vi "FITS - Save a Single I32 Image to FITS.vi"(5 "Neo Info":T1={"Handle"=104, "Pixel Encoding"="Mono16", "AOI Width"=2560, "AOI Height"=2160, "AOI Stride"=5136, "Row Readout Time"=9.371428571428572e-06, "Frame Readout Time"=0.010121142857142858, "Interframe Time"=8.434285714285715e-05, "Semaphore"=refnum, "SerialNumber"="SCC-02209", "Camera Model"="DC-152Q-C00-FI", "Controller ID"="3", "Firmware Version"="13.8.26.122", "Shutter"="Global", "BDiv"=1, "Time at Synch"=timestamp(3029526000.379448 s since 1904-01-01), "Idx"=0, "PreAmp"="", "Binning"=enum."1x1", "PixelReadoutRate"="", "Exposure (s)"=0.05, "Image Bytes"=11098896, "Image Pixels"=5529600, "SpuriousNoiseFilter"=FALSE, "Overlap"=FALSE, "CycleMode"=""} {"Exposure (s)" format="%^.3g"; "Time at Synch" format="%<%H:%M:%S>T"; "Interframe Time" format="%#_3g"; "Frame Readout Time" format="%_3g"; "Row Readout Time" format="%_3g"}, 6 "byte order (0:big-endian, network order)":T4(ring), 7 "FITS Header":T5={"Wavelength (nm)"=530.15, "Exposure (s)"=0.05, "Tuning Delay (ms)"=1000.0, "Beam Type (-1/1)"=1.0, "Tuning Voltages"=[1.111, 2.222, 3.333, 4.444], "Observer"="observer", "Light Shapping Diffuser"=enum."In Beam", "Comment"="", "Data Type"=9, "Mod Cycles"=0, "SCD Calibration Optics"=enum."1 - Polarizer @0, I+Q", "SCD Emission Line Filter"=enum."1-557.6nm", "Cookbook"="", "COMP-S Calibration Wheel"=enum."Dark", "COMP-S Andover Filter Wheel"=enum."530.3nm/HWB 0.34nm (Fe XIV)", "FOV Rotation (deg)"=66.0, "Objective Lens Position (mm)"=0.0, "Occulter size"=0.0, "Time End"=timestamp(3382374145.421875 s since 1904-01-01), "Acc Exposure (s)"=0.0, "Time Stamp Array"=[], "Camera Serial Number"=[], "Camera Temp"=[], "Camera PI (mm)"=[0.0, 0.0, 0.0], "Time Start"=timestamp(3382374145.421875 s since 1904-01-01), "Peripherals"={"ILX controler"=FALSE, "Zone temperatures"=FALSE, "Andor"=FALSE, "Andor 2"=FALSE, "PI Stages"=FALSE, "AISAS mechanisms"=FALSE, "AISAS Mech.lvclass"=refnum, "Zone temp ref"=variant, "FWs"=FALSE}, "FITS paths"=[], "Cameras"=enum."Andor", "load preset cbk"=FALSE, "periodic check count"=0} {"Camera PI (mm)" format="%_3g"; "Acc Exposure (s)" format="%^.3g"; "Occulter size" format="%.2f"; "Objective Lens Position (mm)" min=70.0 max=152.0 format="%.2f"; "FOV Rotation (deg)" format="%.1f"; "Data Type" items=["LIVE", "DARK", "FLAT", "CALI", "OBSE", "ABSO", "AURE", "TARG", "OBJE", "HOLE", "OREX", "THRO", "CHIP"]; "Exposure (s)" format="%^.3g"; "Wavelength (nm)" format="%_6g"}, 8 "error in":errorcluster, 9 "I32 Image Data":i32[](array[numeric]), 10 "Image #":i32, 11 "FITS File Path":path=path "G:/SCD Data/Level-0/20141030/20141030.160747.FTS") -> (0 "error out":errorcluster, 3 "FITS Path Out":path=path "G:/SCD Data/Level-0/20141030/20141030.160747.FTS")   [LabVIEW 2014]
doc: "Duplicate first measurement\nand put it in first element of\nmeasurement array. This\nis a dummy measurement for the\nprimary header. This is because\nwe don't want any images associated\nwith the primary HDU, just the \nextensions. In the Make FITS\nHeaders VI, the NAXIS is set to 0 in\nthis primary HDU"
uses:
  Controls/SCD - FITS Cluster.ctl
  AISAS/Mech/AISAS Mech.lvclass
  AISAS/Controls/Diffuser.ctl
  Controls/SCD - Calibration Optics Filter Wheel.ctl
  Controls/SCD - EDT - Emission Line Filter Wheel.ctl
  Controls/CoMP-S Controls/Polarization Optics Filter Wheel.ctl
  Controls/CoMP-S Controls/Emission Line Filter Wheel.ctl
  AISAS/Controls/focus.ctl
  Controls/peripherals.ctl
  Controls/Cameras select.ctl
  Camera/Andor Neo Info.ctl
  Controls/beaning.ctl
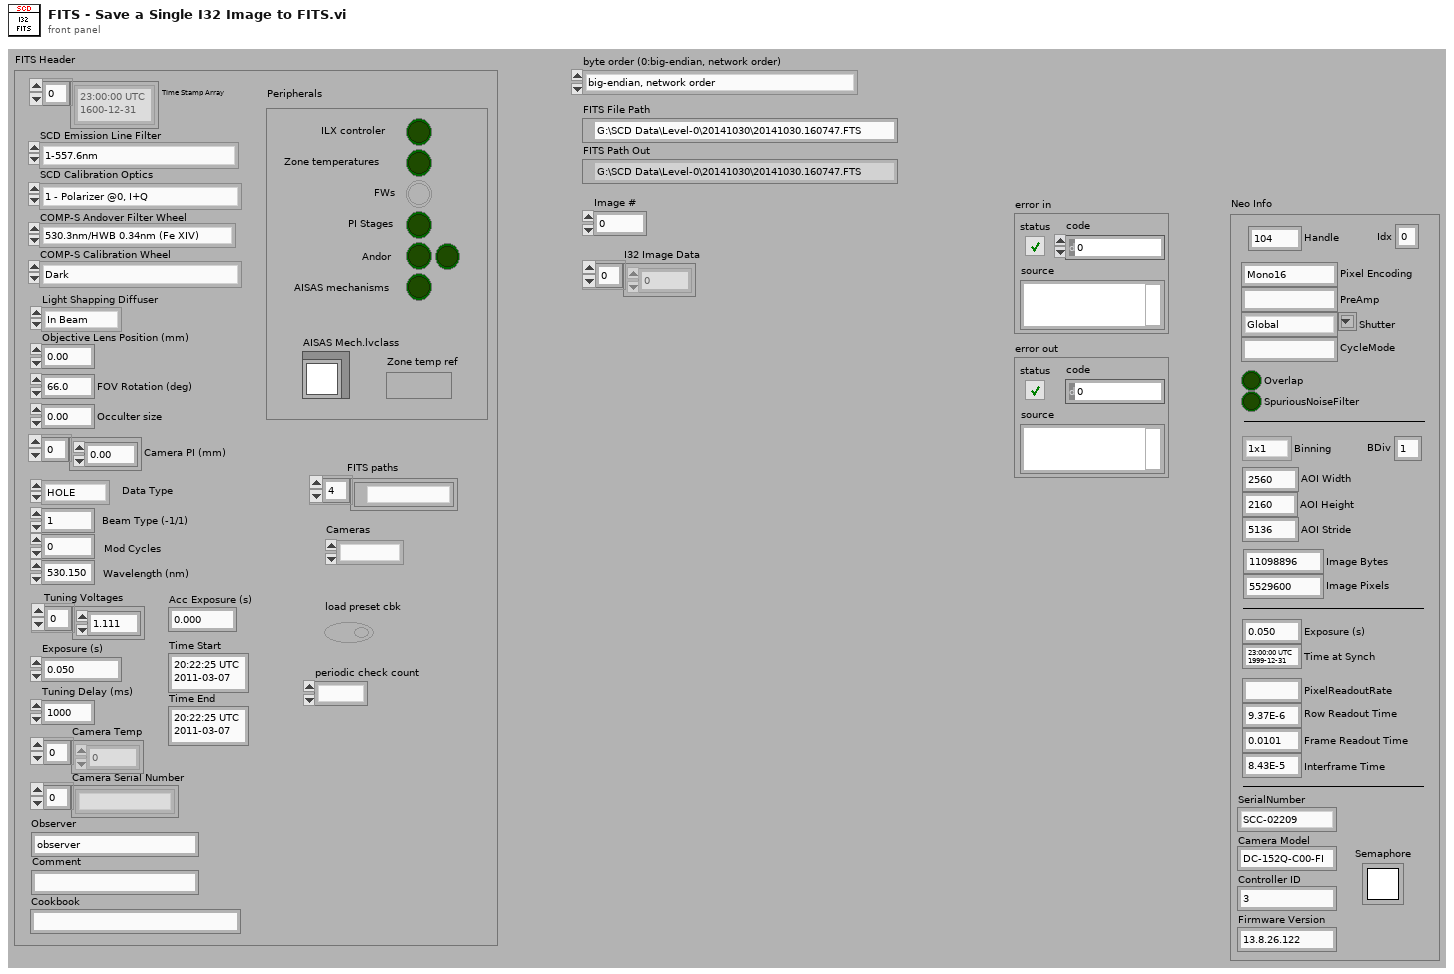
[diagram p1: front panel]
types:
  T1 = typedef "Andor Neo Info.ctl" = cluster{"Handle":i32, "Pixel Encoding":string, "AOI Width":i32, "AOI Height":i32, "AOI Stride":i32, "Row Readout Time":dbl, "Frame Readout Time":dbl, "Interframe Time":dbl, "Semaphore":T2, "SerialNumber":string, "Camera Model":string, "Controller ID":string, "Firmware Version":string, "Shutter":string, "BDiv":u8, "Time at Synch":timestamp, "Idx":i32, "PreAmp":string, "Binning":T3, "PixelReadoutRate":string, "Exposure (s)":dbl, "Image Bytes":i64, "Image Pixels":i64, "SpuriousNoiseFilter":bool, "Overlap":bool, "CycleMode":string}
  T2 = typedef "Semaphore RefNum" = refnum<k1>
  T3 = typedef "beaning.ctl" = enum16{"1x1", "2x2", "3x3", "4x4", "8x8"}
  T4 = enum16{"big-endian, network order", "native, host order", "little-endian"}
  T5 = typedef "SCD - FITS Cluster.ctl" = cluster{"Wavelength (nm)":dbl, "Exposure (s)":dbl, "Tuning Delay (ms)":dbl, "Beam Type (-1/1)":dbl, "Tuning Voltages":dbl[], "Observer":string, "Light Shapping Diffuser":T6, "Comment":string, "Data Type":u16, "Mod Cycles":u16, "SCD Calibration Optics":T7, "SCD Emission Line Filter":T8, "Cookbook":string, "COMP-S Calibration Wheel":T9, "COMP-S Andover Filter Wheel":T10, "FOV Rotation (deg)":dbl, "Objective Lens Position (mm)":T11, "Occulter size":dbl, "Time End":timestamp, "Acc Exposure (s)":dbl, "Time Stamp Array":timestamp[], "Camera Serial Number":string[], "Camera Temp":dbl[], "Camera PI (mm)":dbl[], "Time Start":timestamp, "Peripherals":T12, "FITS paths":path[], "Cameras":T13, "load preset cbk":bool, "periodic check count":i32}
  T6 = typedef "Diffuser.ctl" = enum16{"Out of Beam", "In Beam"}
  T7 = typedef "SCD - Calibration Optics Filter Wheel.ctl" = enum16{"1 - Polarizer @0, I+Q", "2 - Polarizer @90, I-Q", "3 - Polarizer @45, I+U", "4 - Polarizer @135, I-U", "5 - Polarizer @0, Retarder @45, I+V", "6 - Polarizer @0, Retarder @135, I-V", "7 - Dark", "8 - Clear", "9 - N/A"}
  T8 = typedef "SCD - EDT - Emission Line Filter Wheel.ctl" = enum16{"1-557.6nm", "2-587.6nm", "3-589.6nm", "4-630.2nm", "5-656.4nm", "6-849.8nm", "7-854.2nm", "8-866.2nm", "9-1083.0nm"}
  T9 = typedef "Polarization Optics Filter Wheel.ctl" = enum16{"Dark", "Clear", "Exchange Lens", "Polarizer @0, I+Q", "Polarizer @90, I-Q", "Polarizer @45, I+U", "Polarizer @135, I-U", "Polarizer @0, Retarder @45, I+V", "Polarizer @0, Retarder @135, I-V"}
  T10 = typedef "Emission Line Filter Wheel.ctl" = enum16{"530.3nm/HWB 0.34nm (Fe XIV)", "587.6nm/HBW 0.44nm (He I D3)", "637.5nm/HBW 0.53nm (Fe X)", "656.3nm/HBW 0.57nm (H-Alpha)", "789.2nm/HBW 0.85nm (Fe XI)", "854.2nm/HBW 1.01nm (Ca I)", "1074.7nm/HBW 2.34nm (Fe XIII)", "1079.8nm/HBW 1.64nm (Fe XIII)", "1083.0nm/HBW 1.66nm (He I)"}
  T11 = typedef "focus.ctl" = dbl
  T12 = typedef "peripherals.ctl" = cluster{"ILX controler":bool, "Zone temperatures":bool, "Andor":bool, "Andor 2":bool, "PI Stages":bool, "AISAS mechanisms":bool, "AISAS Mech.lvclass":refnum<class "AISAS Mech.lvclass">, "Zone temp ref":variant, "FWs":bool}
  T13 = typedef "Cameras select.ctl" = enum16{"Andor", "GDR"}
  T14 = enum16{"open", "replace", "create", "open or create", "replace or create", "replace or create with confirmation"}
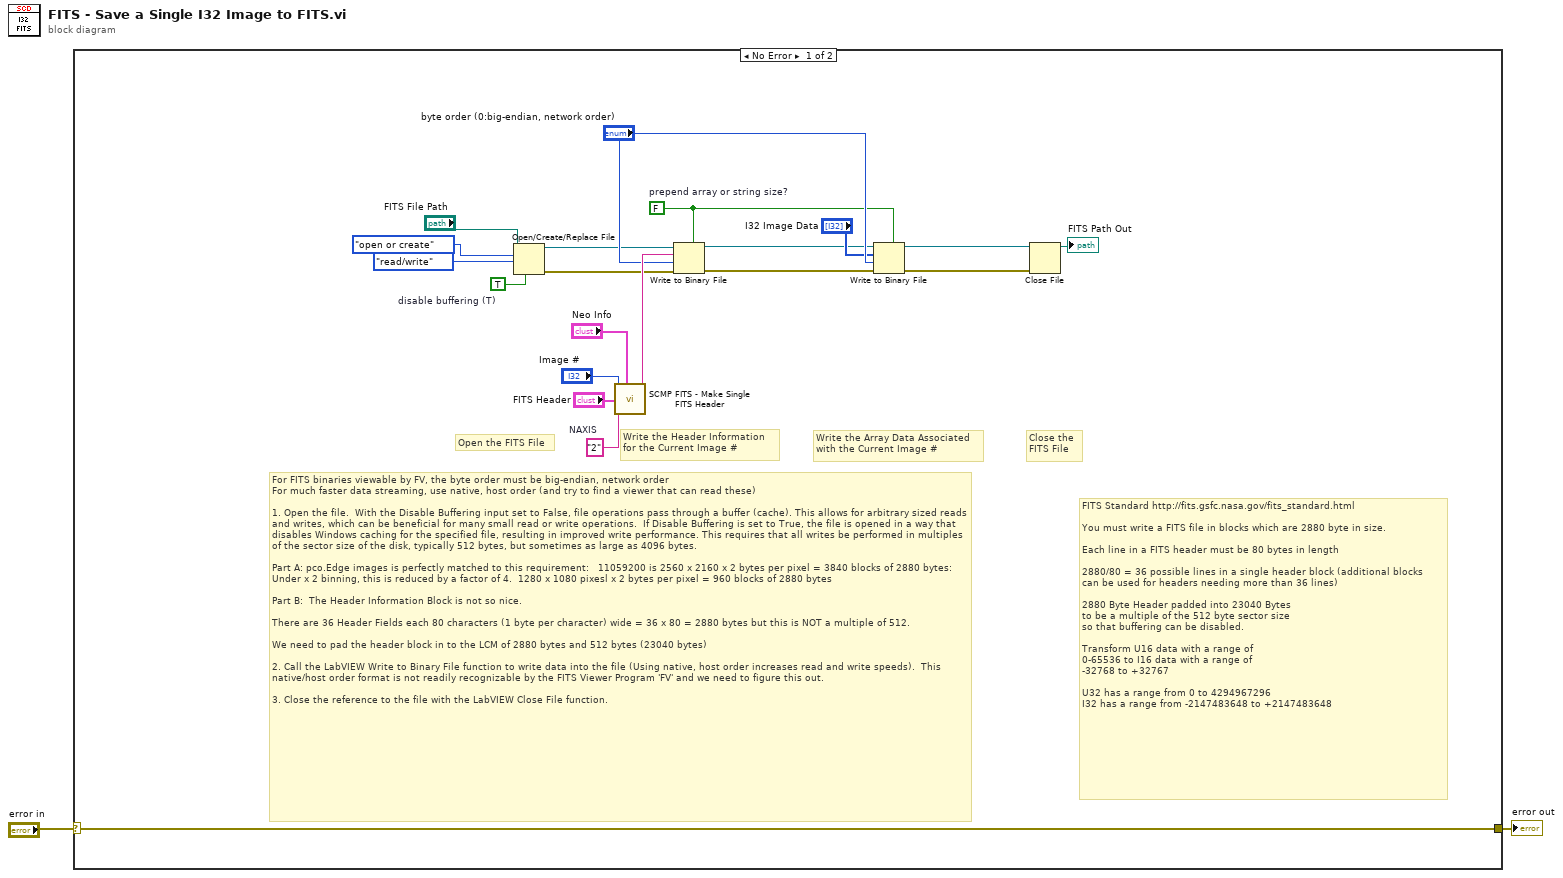
[diagram p0: block diagram]
diagram:
  n1 = case shown="No Error" "error in" {
    selector: "error in" -> [w13 w23]
    tunnel: [w13 w23] -> w1
    frame No Error {
      w4 = "2"  # NAXIS
      w5 = FALSE  # prepend array or string size?
      w15 = TRUE  # disable buffering (T)
      # "FITS Standard http://fits.gsfc.nasa.gov/fits_standard.html\n\nYou must write a FITS file in blocks which are 2880 byte in size.\n\nEach line in a FITS header must be 80 bytes in length\n\n2880/80 = 36 possible lines in a single header block (additional blocks\ncan be used for headers needing more than 36 lines)\n\n2880 Byte Header padded into 23040 Bytes\nto be a multiple of the 512 byte sector size\nso that buffering can be disabled.\n\nTransform U16 data with a range of\n0-65536 to I16 data with a range of\n-32768 to +32767\n\nU32 has a range from 0 to 4294967296\nI32 has a range from -2147483648 to +2147483648"
      # "For FITS binaries viewable by FV, the byte order must be big-endian, network order\nFor much faster data streaming, use native, host order (and try to find a viewer that can read these)\n\n1. Open the file.  With the Disable Buffering input set to False, file operations pass through a buffer (cache). This allows for arbitrary sized reads and writes, which can be beneficial for many small read or write operations.  If Disable Buffering is set to True, the file is opened in a way that disables Windows caching for the specified file, resulting in improved write performance. This requires that all writes be performed in multiples of the sector size of the disk, typically 512 bytes, but sometimes as large as 4096 bytes.\n\nPart A: pco.Edge images is perfectly matched to this requirement:   11059200 is 2560 x 2160 x 2 bytes per pixel = 3840 blocks of 2880 bytes:  Under x 2 binning, this is reduced by a factor of 4.  1280 x 1080 pixesl x 2 bytes per pixel = 960 blocks of 2880 bytes\n\nPart B:  The Header Information Block is not so nice.  \n\nThere are 36 Header Fields each 80 characters (1 byte per character) wide = 36 x 80 = 2880 bytes but this is NOT a multiple of 512.\n\nWe need to pad the header block in to the LCM of 2880 bytes and 512 bytes (23040 bytes)\n\n2. Call the LabVIEW Write to Binary File function to write data into the file (Using native, host order increases read and write speeds).  This native/host order format is not readily recognizable by the FITS Viewer Program 'FV' and we need to figure this out.\n\n3. Close the reference to the file with the LabVIEW Close File function."
      # "Close the \nFITS File"
      # "Write the Array Data Associated\nwith the Current Image #"
      # "Write the Header Information\nfor the Current Image #"
      # "Open the FITS File"
      n2 = Open/Create/Replace File(file path (use dialog)="FITS File Path", operation (0:open)=T14."open or create", access (0:read/write)=enum16{"read/write", "read-only", "write-only"}."read/write", disable buffering (F)=w15) -> (refnum out=w7:refnum<file>, error out=w8:errorcluster)  [unwired: 1 in, 2 out]
      n3 = call "SCMP FITS - Make Single FITS Header.vi"("Andor"="Neo Info", "NAXIS"=w4, "FITS Header"="FITS Header", "Image #"="Image #") -> ("23040 Byte Header"=w14:string)  [unwired: 3 in, 4 out]
      n4 = Write to Binary File(file (use dialog)=w7, data=w14, error in=w8, 5:w5, 9:"byte order (0:big-endian, network order)") -> (refnum out=w6:refnum<file>, error out=w9:errorcluster)  [unwired: 2 out]
      n5 = Write to Binary File(file (use dialog)=w6, data="I32 Image Data", error in=w9, 5:w5, 9:"byte order (0:big-endian, network order)") -> (refnum out=w21:refnum<file>, error out=w22:errorcluster)  [unwired: 2 out]
      n6 = Close File(refnum=w21, error in=w22) -> (path=→"FITS Path Out":path)  [unwired: 1 out]
    }
    frame Error {
    }
  }
  "error out" <- w1
